vi "niVNA_FrequencyOffset_Mod.vi"() -> ()   [LabVIEW 2013]
uses:
  <instrlib>/niVNA/niVNA.llb/niVNA Fetch Receiver Measurement Complex (CDB).vi
  <instrlib>/niVNA/niVNA.llb/niVNA Load Calibration And Configuration Data From File.vi
  <instrlib>/niVNA/niVNA.llb/niVNA Configure Frequency Start Stop.vi
  <instrlib>/niVNA/niVNA.llb/niVNA Fetch Sweep Measurement Complex (CDB).vi
panel:
  out "CPD@ offset?":dbl[](graph)
  out "CPD 2":dbl[](graph)
  in  "Number of points":i32=201
  in  "stop frequency":dbl=4200000000.0 format="%#_6p"
  in  "start frequency":dbl=3800000000.0 format="%#_6p"
  in  "SavedCalPath":path=path "C:/Users/Eddie.Rickey/Documents/RCV_PXI/Calibration/#Cal - VNA_ 50MHz_mod.chx"
  in  "Port2 Source Driving State":i32(ring) items=["Automatic", "Active", "Inactive"]
  in  "Receivers Frequency Offset":dbl=100000000.0 format="%#_6p"
  in  "Receivers Frequency Multiplier":dbl=1.0
  in  "Port2 Frequency Offset":dbl=4100000000.0 format="%#_6p"
  in  "Port1 Source Driving State":i32(ring) items=["Automatic", "Active", "Inactive"]
  in  "Port2 Frequency Multiplier":dbl
  in  "Port1 Frequency Multiplier":dbl
  in  "Port1 Frequency Offset":dbl=4000000000.0 format="%#_6p"
  in  "stop":bool
  out "error out":errorcluster
  in  "receiver port":string(combo)="port2"
  in  "receiver port":string(combo)="port1"
  in  "driving port":string(combo)="port1"
  in  "receiver":i32(ring)=10 items=["Test Receiver"=10, "Reference Receiver"=11]
  in  "format":i32(ring) items=["Log Magnitude (dB)"=0, "Lin Magnitude"=1, "Phase (deg)"=2, "VSWR"=3, "Group Delay"=6]
  in  "receiver":i32(ring)=11 items=["Test Receiver"=10, "Reference Receiver"=11]
  out "XY Graph 2":cluster{"scale points":dbl[], "data":dbl[]}(graph)
  in  "format":i32(ring) items=["Log Magnitude (dB)"=0, "Lin Magnitude"=1, "Phase (deg)"=2, "VSWR"=3, "Group Delay"=6]
  in  "resource name":refnum<k15>="PXI1Slot2"
  out "XY Graph":cluster{"scale points":dbl[], "data":dbl[]}(graph)
  # "This VI shows the how to use frequency offsets\nfor the source and receiver in NI-VNA.\n\nInstructions:\n1. Select device in resource name.\n2. Configure sweep parameters.\n3. Run the VI.\n4. Select output display parameters."
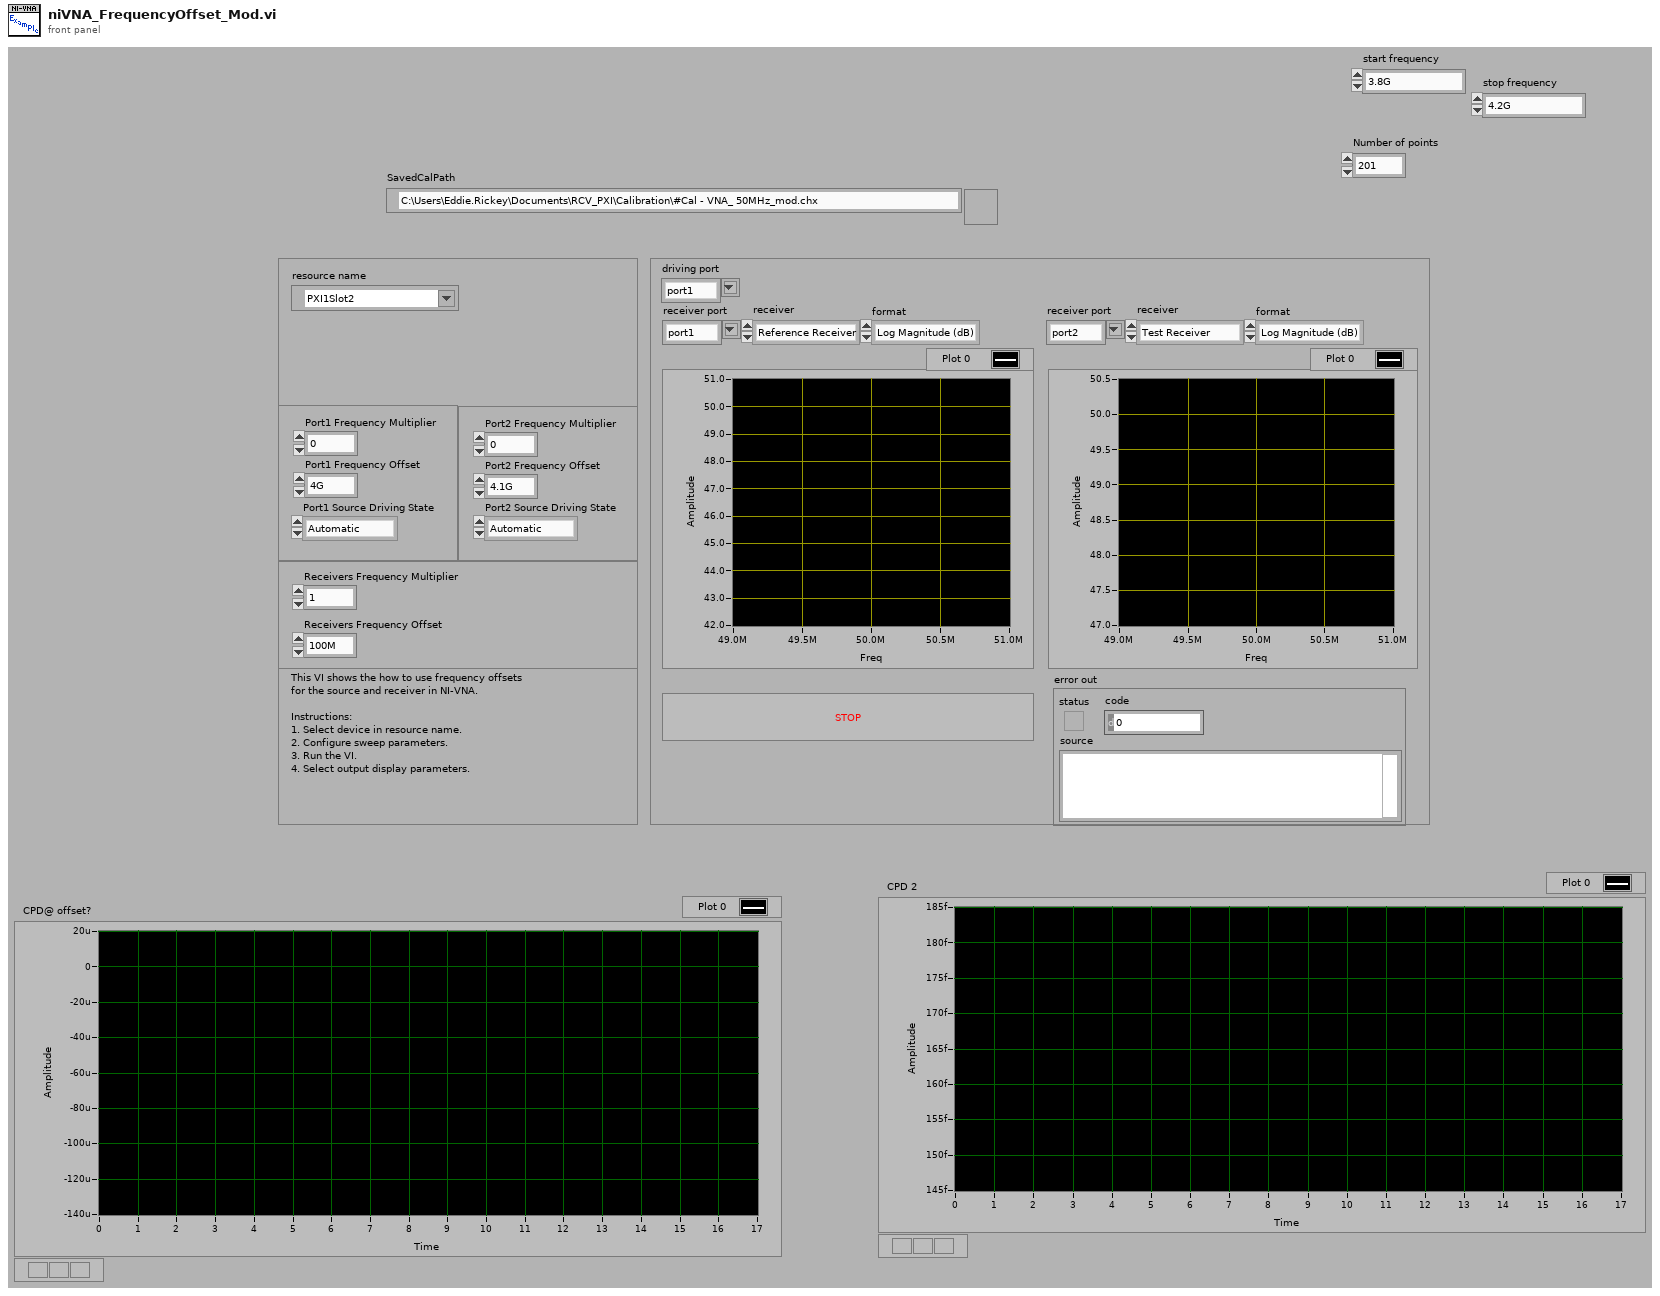
[diagram p1: front panel]
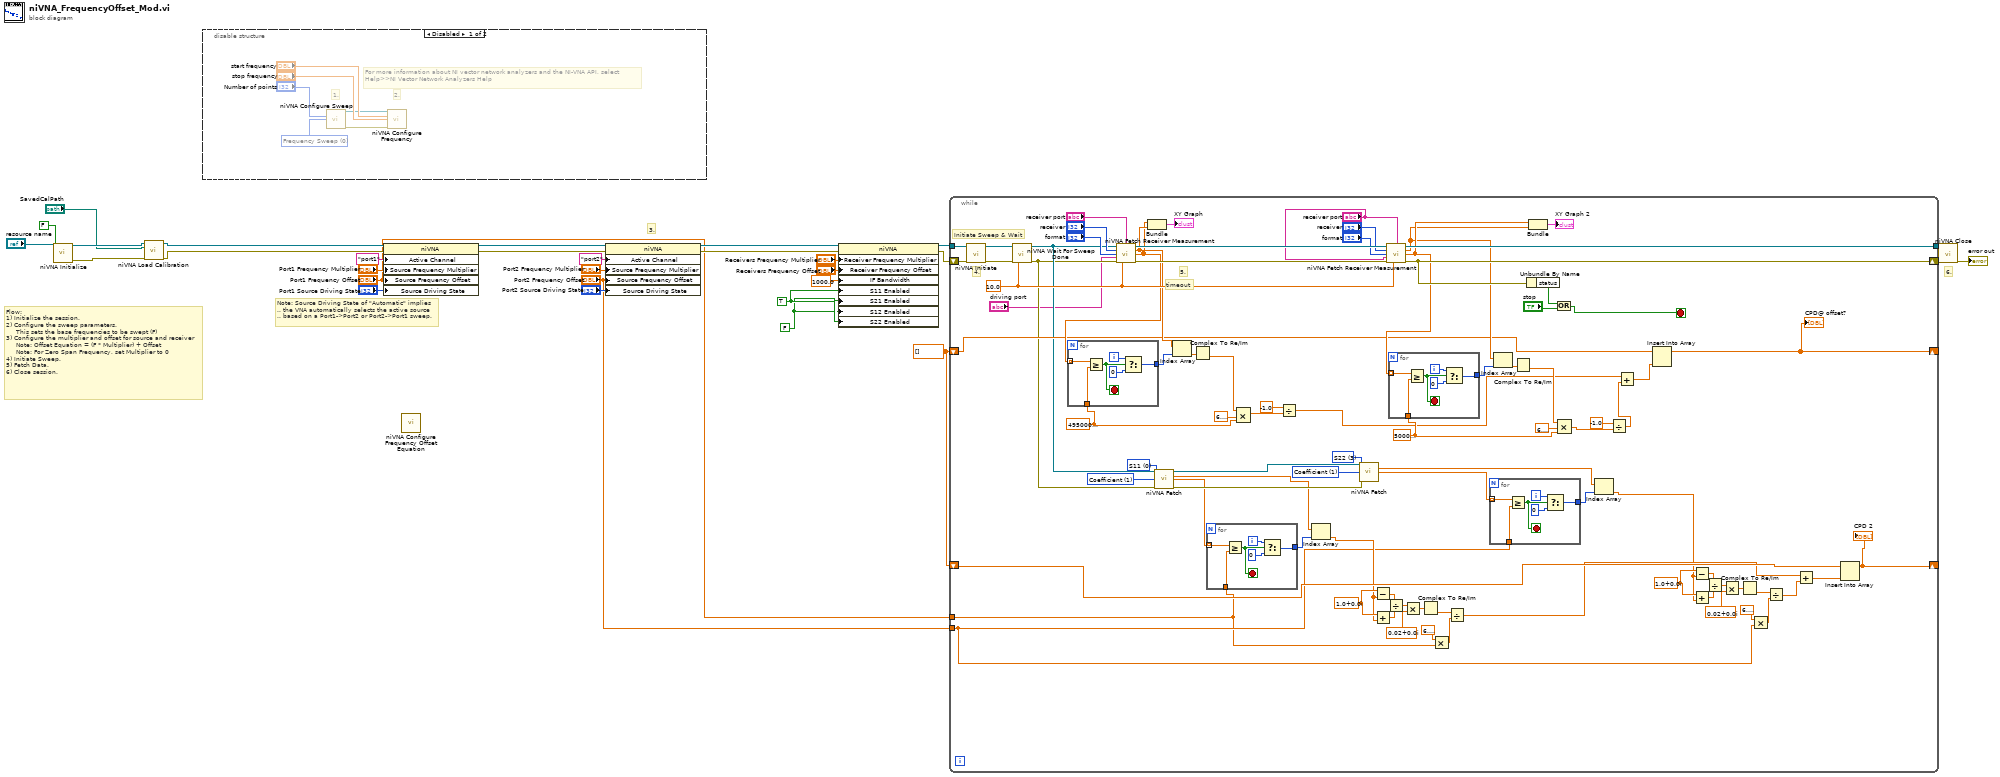
[diagram p0: block diagram]
diagram:
  w3 = FALSE ("Sweep:S11 Enabled")
  w4 = TRUE ("Sweep:S11 Enabled")
  w5 = dbl[] []
  # "Note: Source Driving State of \"Automatic\" implies\n.. the VNA automatically selects the active source \n.. based on a Port1->Port2 or Port2->Port1 sweep."
  # "6."
  # "3."
  # "Flow:\n1) Initialize the session.\n2) Configure the sweep parameters.\n     This sets the base frequencies to be swept (F)\n3) Configure the multiplier and offset for source and receiver\n     Note: Offset Equation = (F * Multiplier) + Offset\n     Note: For Zero Span Frequency, set Multiplier to 0\n4) Initiate Sweep.\n5) Fetch Data.\n6) Close session."
  n1 = call <instrlib>:"niVNA Initialize.vi"("resource name"="resource name", "reset"=FALSE) -> ("instrument handle"=w9:refnum<k15>, "error out"=w10:errorcluster)  [unwired: 2 in, 10 out]
  n2 = call-poly <instrlib>:"niVNA Load Calibration.vi"("instrument handle"=w9, "file path"="SavedCalPath", "error in"=w10) -> ("instrument handle out"=w8:refnum<k15>, "error out"=w7:errorcluster)  [unwired: 11 in]
  n3 = disable-structure shown="Disabled" {
    frame Disabled {
      w35 = 0 items=["Frequency Sweep", "Power Sweep"] ("sweep mode")
      # "2."
      # "1."
      # "For more information about NI vector network analyzers and the NI-VNA API, select\nHelp>>NI Vector Network Analyzers Help"
      n4 = call <instrlib>:"niVNA Configure Sweep.vi"("number of points"="Number of points", "sweep mode"=w35) -> ("instrument handle"=w37:refnum<k15>, "instrument handle out"=w33:refnum<k15>, "error in"=w34:errorcluster, "error out"=w32:errorcluster)  [unwired: 10 in]
      n5 = call-poly <instrlib>:"niVNA Configure Frequency.vi"("instrument handle"=w33, "start frequency"="start frequency", "stop frequency"="stop frequency", "error in"=w32) -> ("error out"=w31:errorcluster)  [unwired: 1 in, 10 out]
    }
    frame Enabled {
    }
  }
  n6 = property class="niVNA"(reference=w8, error in=w7, "Active Channel"="port1", "Source Frequency Multiplier"="Port1 Frequency Multiplier", "Source Frequency Offset"="Port1 Frequency Offset", "Source Driving State"="Port1 Source Driving State") -> (reference out=w22:refnum<k15>, error out=w21:errorcluster)
  n7 = call <instrlib>:"niVNA Configure Frequency Offset Equation.vi"() -> ()  [unwired: 14 in, 2 out]
  n8 = property class="niVNA"(reference=w22, error in=w21, "Active Channel"="port2", "Source Frequency Multiplier"="Port2 Frequency Multiplier", "Source Frequency Offset"="Port2 Frequency Offset", "Source Driving State"="Port2 Source Driving State") -> (reference out=w20:refnum<k15>, error out=w19:errorcluster)
  n9 = property class="niVNA"(reference=w20, error in=w19, "Receiver Frequency Multiplier"="Receivers Frequency Multiplier", "Receiver Frequency Offset"="Receivers Frequency Offset", "IF Bandwidth"=1000.0 ("Test Signal:Output Power"), "S11 Enabled"=w4, "S21 Enabled"=w3, "S12 Enabled"=w3, "S22 Enabled"=w4) -> (reference out=w16:refnum<k15>, error out=w15:errorcluster)
  n10 = while {
    tunnel: w16 -> [w120]
    tunnel: [w117] -> w29
    shift-right: [w107] -> w28
    shift-left: w15 -> [w106]
    shift-right: [w41] -> _
    shift-left: w5 -> [w92]
    shift-right: [w50] -> _
    shift-left: w5 -> [w51]
    tunnel: "Port2 Frequency Offset" -> [w44]
    tunnel: "Port1 Frequency Offset" -> [w43]
    stop <- w110 stop-if-true
    w60 = cdb 1.0+0.0i
    w69 = cdb 1.0+0.0i
    w78 = 1 items=["Impedance", "Coefficient"] ("format")
    w79 = 3 items=["S11", "S21", "S12", "S22"] ("measurement")
    w80 = 1 items=["Impedance", "Coefficient"] ("format")
    w81 = 0 items=["S11", "S21", "S12", "S22"] ("measurement")
    w97 = 50000000.0 ("element")
    w101 = 49500000.0 ("element")
    w112 = 10.0 ("timeout")
    # "5."
    # "4."
    # "timeout"
    # "Initiate Sweep & Wait"
    n11 = call <instrlib>:"niVNA Initiate.vi"("instrument handle"=w120, "error in"=w106) -> ("instrument handle out"=w124:refnum<k15>, "error out"=w123:errorcluster)  [unwired: 12 out]
    n12 = call <instrlib>:"niVNA Wait For Sweep Done.vi"("instrument handle"=w124, "error in"=w123, "timeout"=w112) -> ("instrument handle out"=w83:refnum<k15>, "error out"=w82:errorcluster)  [unwired: 11 out]
    n13 = call-poly <instrlib>:"niVNA Fetch Receiver Measurement.vi"("instrument handle"=w83, "receiver port"="receiver port", "receiver"="receiver", "format"="format", "driving port"="driving port", "error in"=w82, "timeout"=w112) -> ("instrument handle out"=w118:refnum<k15>, "data"=w105:cdb[], "scale points"=w102:dbl[], "error out"=w116:errorcluster)  [unwired: 5 in]
    n14 = for {
      tunnel: w102 -> [w148] mode=indexing
      tunnel: w101 -> [w147]
      tunnel: [w143] -> w100
      i -> [w146]
      stop <- w145 stop-if-true
      n15 = Greater Or Equal?(x=w148, y=w147) -> (x >= y?=w145:bool)
      n16 = Select(t=w146, s=w145, f=0) -> (s? t:f=w143:i32)
    }
    n17 = Bundle("scale points"=w102, "data"=w105) -> (→"XY Graph":cluster{"scale points":dbl[], "data":cdb[]})  [unwired: 1 out]
    n18 = call-poly <instrlib>:"niVNA Fetch.vi"("instrument handle"=w83, "measurement"=w81, "format"=w80, "error in"=w82) -> ("instrument handle out"=w77:refnum<k15>, "data"=w73:cdb[], "scale points"=w74:dbl[], "error out"=w76:errorcluster)  [unwired: 8 in]
    n19 = Index Array(array=w105, index=w100) -> (element=w104:cdb)
    n20 = Complex To Re/Im(x + iy=w104) -> (y=w91:dbl)  [unwired: 1 out]
    n21 = for {
      tunnel: w74 -> [w136] mode=indexing
      tunnel: w43 -> [w135]
      tunnel: [w131] -> w75
      i -> [w134]
      stop <- w133 stop-if-true
      n22 = Greater Or Equal?(x=w136, y=w135) -> (x >= y?=w133:bool)
      n23 = Select(t=w134, s=w133, f=0) -> (s? t:f=w131:i32)
    }
    n24 = Compound Arithmetic op=MULTIPLY(w91, 6.283185307179586, w101) -> (w90:dbl)
    n25 = Divide(x=-1.0, y=w90) -> (x/y=w84:dbl)
    n26 = Index Array(array=w73, index=w75) -> (element=w46:cdb)
    n27 = call-poly <instrlib>:"niVNA Fetch.vi"("instrument handle"=w77, "measurement"=w79, "format"=w78, "error in"=w76) -> ("data"=w70:cdb[], "scale points"=w71:dbl[])  [unwired: 8 in, 2 out]
    n28 = Subtract(x=w69, y=w46) -> (x-y=w68:cdb)
    n29 = Add(x=w69, y=w46) -> (x+y=w67:cdb)
    n30 = call-poly <instrlib>:"niVNA Fetch Receiver Measurement.vi"("instrument handle"=w118, "receiver port"="receiver port", "receiver"="receiver", "format"="format", "driving port"="receiver port", "error in"=w116, "timeout"=w112) -> ("instrument handle out"=w117:refnum<k15>, "data"=w94:cdb[], "scale points"=w95:dbl[], "error out"=w107:errorcluster)  [unwired: 5 in]
    n31 = Divide(x=w68, y=w67) -> (x/y=w66:cdb)
    n32 = for {
      tunnel: w95 -> [w142] mode=indexing
      tunnel: w97 -> [w141]
      tunnel: [w137] -> w96
      i -> [w140]
      stop <- w139 stop-if-true
      n33 = Greater Or Equal?(x=w142, y=w141) -> (x >= y?=w139:bool)
      n34 = Select(t=w140, s=w139, f=0) -> (s? t:f=w137:i32)
    }
    n35 = Multiply(x=w66, y=cdb 0.02+0.0i) -> (x*y=w64:cdb)
    n36 = Complex To Re/Im(x + iy=w64) -> (y=w62:dbl)  [unwired: 1 out]
    n37 = Multiply(x=6.283185307179586, y=w43) -> (x*y=w61:dbl)
    n38 = Divide(x=w62, y=w61) -> (x/y=w48:dbl)
    n39 = for {
      tunnel: w71 -> [w130] mode=indexing
      tunnel: w44 -> [w129]
      tunnel: [w125] -> w72
      i -> [w128]
      stop <- w127 stop-if-true
      n40 = Greater Or Equal?(x=w130, y=w129) -> (x >= y?=w127:bool)
      n41 = Select(t=w128, s=w127, f=0) -> (s? t:f=w125:i32)
    }
    n42 = Index Array(array=w94, index=w96) -> (element=w99:cdb)
    n43 = Complex To Re/Im(x + iy=w99) -> (y=w88:dbl)  [unwired: 1 out]
    n44 = Unbundle By Name(w107) -> ("status"=w108:bool)
    n45 = Bundle("scale points"=w95, "data"=w94) -> (→"XY Graph 2":cluster{"scale points":dbl[], "data":cdb[]})  [unwired: 1 out]
    n46 = Or(x=w108, y="stop") -> (x .or. y?=w110:bool)
    n47 = Compound Arithmetic op=MULTIPLY(w88, 6.283185307179586, w97) -> (w86:dbl)
    n48 = Index Array(array=w70, index=w72) -> (element=w45:cdb)
    n49 = Divide(x=-1.0, y=w86) -> (x/y=w85:dbl)
    n50 = Add(x=w84, y=w85) -> (x+y=w93:dbl)
    n51 = Insert Into Array(array=w92, new element=w93) -> (w41:dbl[])  [unwired: 1 in]
    "CPD@ offset?" <- w41
    n52 = Subtract(x=w60, y=w45) -> (x-y=w59:cdb)
    n53 = Add(x=w60, y=w45) -> (x+y=w58:cdb)
    n54 = Divide(x=w59, y=w58) -> (x/y=w57:cdb)
    n55 = Multiply(x=w57, y=cdb 0.02+0.0i) -> (x*y=w55:cdb)
    n56 = Complex To Re/Im(x + iy=w55) -> (y=w53:dbl)  [unwired: 1 out]
    n57 = Multiply(x=6.283185307179586, y=w44) -> (x*y=w52:dbl)
    n58 = Divide(x=w53, y=w52) -> (x/y=w47:dbl)
    n59 = Add(x=w48, y=w47) -> (x+y=w49:dbl)
    n60 = Insert Into Array(array=w51, new element=w49) -> (w50:dbl[])  [unwired: 1 in]
    "CPD 2" <- w50
  }
  n61 = call <instrlib>:"niVNA Close.vi"("instrument handle"=w29, "error in"=w28) -> ("error out"=→"error out":errorcluster)  [unwired: 13 out]
